vi "Dashboard Main.vi"() -> ()   [LabVIEW 2020]
uses:
  <vilib>/event_ctls.llb/eventvkey.ctl
  <vilib>/Rock Robotics/Network Tables/NT Read Numeric Array.vi
  <vilib>/Rock Robotics/WPI/Dashboard/WPI_DashboardLogging Global.vi
  <vilib>/Rock Robotics/Network Tables/NT Read Boolean.vi
  <vilib>/Rock Robotics/Network Tables/NT Write Boolean.vi
panel:
  in  "Camera Settings Right":T1={"Frame Rate"=30, "Compression"=30, "Size"=1, "DB Camera Config"=FALSE} {"Frame Rate" scale=1.0..30.0; "Compression" scale=100.0..-1.0; "Size" items=["640x480", "320x240", "160x120"]}
  in  "Camera Name Right":string(combo)="No Camera Selection"
  out "Camera Perf":string
  in  "Camera Settings":T1={"Frame Rate"=30, "Compression"=30, "Size"=1, "DB Camera Config"=FALSE} {"Frame Rate" scale=1.0..30.0; "Compression" scale=100.0..-1.0; "Size" items=["640x480", "320x240", "160x120"]}
  in  "TCP":refnum<k5>
  in  "Rec Mode":enum32{"Stop", "Record", "Playback"}(radio)
  out "Robot IP":string
  out "Image Message":string="Timeout in Camera Communications"
  in  "Dashboard Tab":T2(tab)=enum."Custom"
  in  "Select Auto":string(combo)="Select Autonomous ..."
  out "NT Connection":bool
  out "MotorChart R":cluster{"Numeric":dbl, "Numeric":dbl}(graph)
  out "MotorChart L":cluster{"Numeric":dbl, "Numeric":dbl}(graph)
  out "MotorSliders R":cluster{"MotorSlide1":dbl, "MotorSlide2":dbl} {"MotorSlide2" scale=-1.0..1.0 scale format="%#_2e"; "MotorSlide1" scale=-1.0..1.0 scale format="%#_2e"}
  out "MotorSliders L":cluster{"MotorSlide1":dbl, "MotorSlide2":dbl} {"MotorSlide2" scale=-1.0..1.0 scale format="%#_2e"; "MotorSlide1" scale=-1.0..1.0 scale format="%#_2e"}
  out "Gyro":dbl(knob) scale=0.0..360.0
  out "JS1 Z":dbl(slide) scale=-1.0..1.0 scale format="%#_2e"
  out "JS1 Graph":cluster{"X":dbl, "Y":dbl}[](graph)
  out "JS1 Buttons":T3
  out "JS2 Z":dbl(slide) scale=-1.0..1.0 scale format="%#_2e"
  out "JS2 Graph":cluster{"X":dbl, "Y":dbl}[](graph)
  out "JS2 Buttons":T3
  out "Mode":T4(ring)=enum."Auto Disabled"
  out "Right Camera Perf":cluster{"Bandwidth (Mbps)":dbl, "FPS":dbl}
  out "Camera Image Right":T5(plugin-control)
  in  "DB/String 9":string
  in  "DB/String 8":string
  in  "DB/String 7":string
  in  "DB/String 6":string
  in  "DB/String 5":string
  in  "DB/String 4":string
  in  "DB/String 3":string
  in  "DB/String 2":string
  in  "DB/String 1":string
  in  "DB/String 0":string
  in  "DB/Slider 0":dbl(slide) scale=0.0..5.0
  in  "DB/Slider 1":dbl(slide) scale=0.0..5.0
  in  "DB/Slider 2":dbl(slide) scale=0.0..5.0
  in  "DB/Slider 3":dbl(slide) scale=0.0..5.0
  out "DB/LED 3":bool
  out "DB/LED 2":bool
  out "DB/LED 1":bool
  out "DB/LED 0":bool
  in  "DB/Button 3":bool
  in  "DB/Button 2":bool
  in  "DB/Button 1":bool
  in  "DB/Button 0":bool caption="New Name"
  in  "Y2":dbl
  in  "Y1":dbl
  in  "X2":dbl
  in  "X1":dbl
  in  "BasicSpool":dbl
  in  "BasicArm":dbl
  in  "DforTSpeed":dbl
  in  "MobilityD":dbl
  in  "True = facing nodes\nFalse = not":bool=TRUE
  in  "Hybrid":bool
  in  "Mobility?":bool
  in  "Cone?":bool
  in  "offset":dbl
  in  "True = High\nFalse = Low":bool
  in  "Node#":dbl
  in  "True = Blue\nFalse  = Red":bool
  out "Transmit FiFo count":dbl
  out "BusOffCount":dbl
  out "Transmit Err":dbl
  out "Err count":dbl
  out "Util%":dbl
  in  "Auto Delay":dbl
  out "Back right":dbl
  out "Back left":dbl
  out "Front right":dbl
  out "Front left":dbl
  out "Navx connected":bool
  out "yaw":dbl
  in  "Test Slider":dbl(slide) scale=0.0..100.0 scale format="%#_3g"
  in  "On/Off":bool caption="Solenoid"
  in  "Test Name":u16(ring) items=["Select the test to run..."]
  in  "Test Tree":string(tree)
  in  "Motor":cluster{"Value":dbl, "Enable":bool} {"Value" scale=-1.0..1.0 scale format="%#_3g"}
  out "Progress":T6 {"Test Progress" scale=0.0..100.0}
  in  "Rev/Fwd":cluster{"Forward":bool, "Reverse":bool}
  in  "Test Ring":u16(ring) items=["Monochrome", "Color"]
  in  "CheckList":i32(listbox)
  out "Tree":string(tree)
  out "Camera Image":T5(plugin-control)
  out "Background":bool
  in  "Camera Name":string(combo)="No Camera Selection"
  # "HW"
  # "HW"
  # "Joysticks"
  # "Drive Motors"
  # "Front"
  # "Right"
  # "Left"
  # "Back"
  # "AUTO"
  # "CAN stuff"
  # "POINTS FOR PLOTPURSUIT"
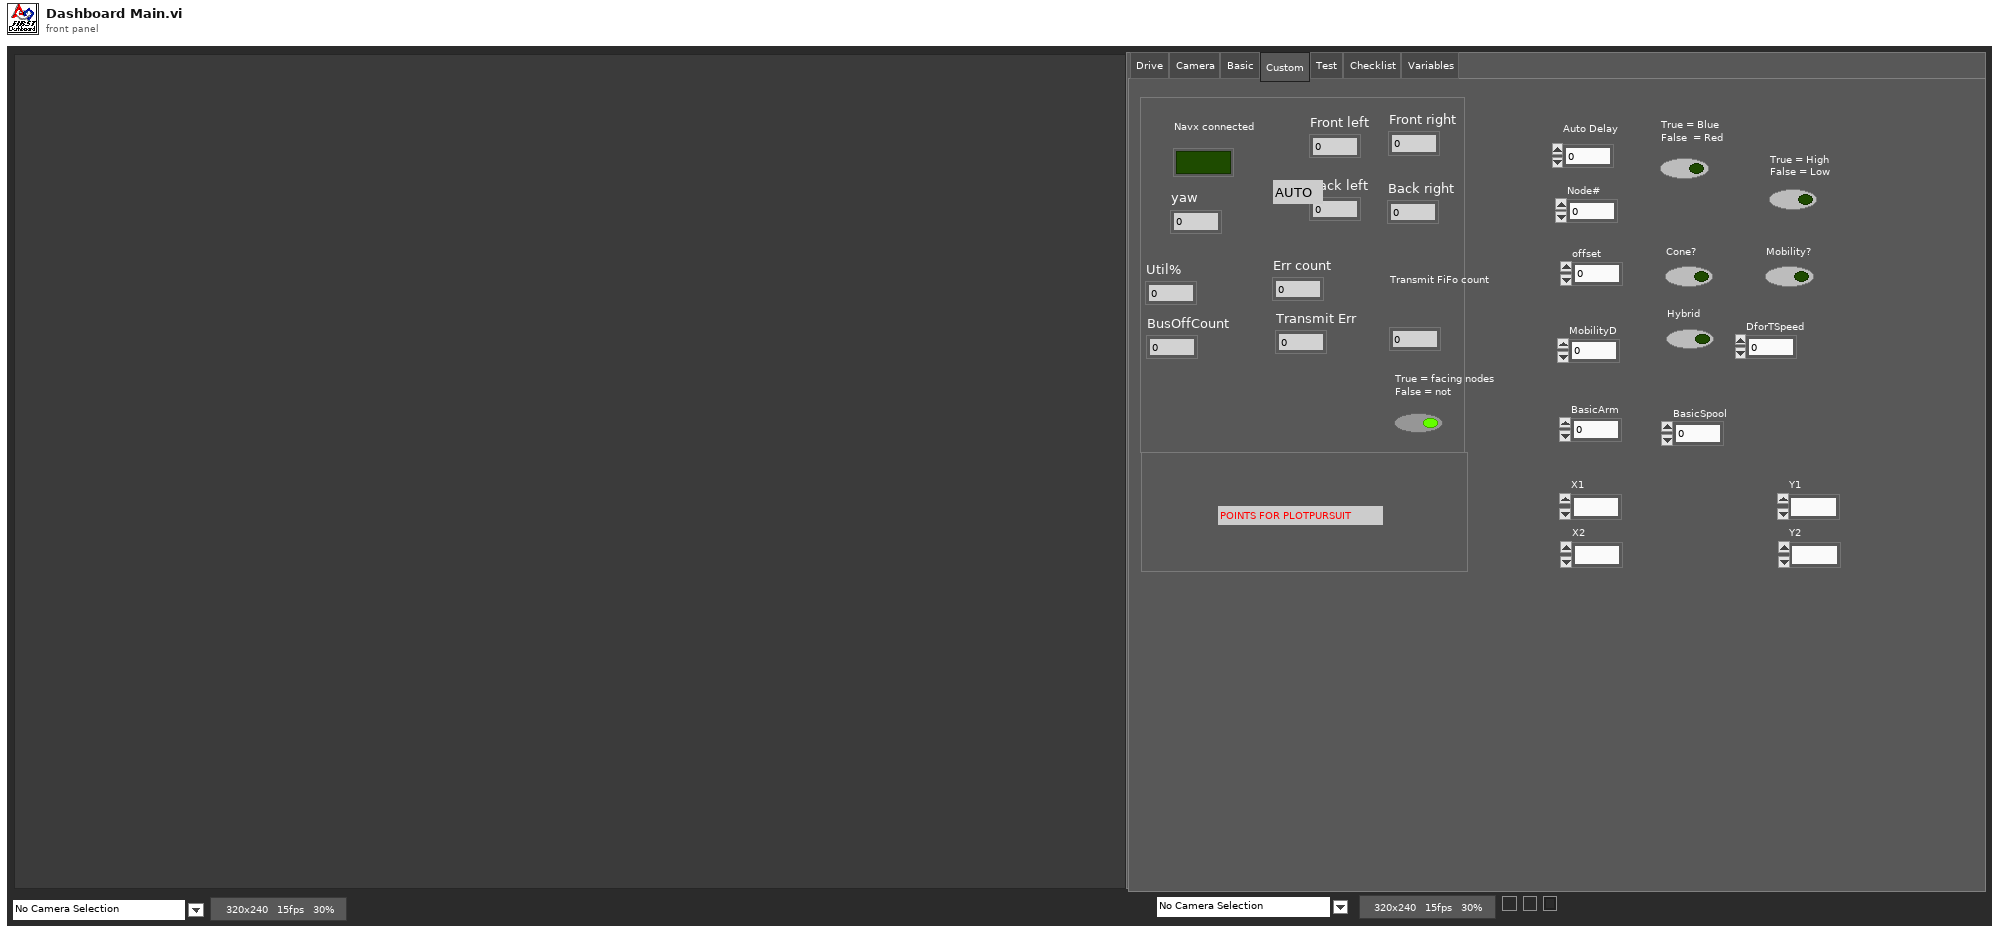
[diagram p1: front panel]
types:
  T1 = cluster{"Frame Rate":i32, "Compression":i32, "Size":u16, "DB Camera Config":bool}
  T2 = enum32{"Drive", "Camera", "Basic", "Custom", "Test", "Checklist", "Variables"}
  T3 = cluster{bool, bool, bool, bool, bool, bool, bool, bool, bool, bool, bool, bool}
  T4 = enum8{"Tele-Op Disabled", "Tele-Op Enabled", "Auto Disabled", "Auto Enabled", "Test Disabled", "Test Enabled", "Disconnected", "No Code", "E-Stop"}
  T5 = typedef "IMAQ Image.ctl" = refnum<image>
  T6 = cluster{"Test Progress":u8, "Test Progress Text":string}
  T7 = cluster{"Save Path":path, "Interval (s)":dbl, "Keep":i32}
  T8 = enum32{"Drive", "Camera", "Basic", "Custom", "Test", "Commands", "Checklist", "Variables"}
  T9 = typedef "Image Type" = u32
  T10 = cluster{"Camera Image":refnum<vi>, "Dashboard Tab":refnum<vi>, "Background":refnum<vi>, "Rec Mode":refnum<vi>, "Test Slider":refnum<vi>, "On/Off ":refnum<vi>, "Test Ring":refnum<vi>, "Rev/Fwd":refnum<vi>, "Test Name":refnum<vi>, "Motor":refnum<vi>, "Progress":refnum<vi>, "CheckList":refnum<vi>, "Tree":refnum<vi>, "Test Tree":refnum<vi>, "Camera Settings":refnum<vi>, "Camera Name":refnum<vi>, "Camera Perf":refnum<vi>, "Camera Settings Right":refnum<vi>, "Camera Name Right":refnum<vi>, "Camera Image Right":refnum<vi>}
  T11 = cluster{"Global Rectangle":i32[], "Contours":cluster{"Contour Type":u32, "ROI Type":u32, "Points":i32[]}[]}
  T12 = cluster{"Camera Name Right":string, string, "Saved DB Images Info":cluster{"Save Path":path, "Interval (s)":dbl, "Keep":i32}}
  T13 = cluster{"Operation":enum16{"Update", "Clear"}, "Color Box":u32}[]
  T14 = typedef "eventvkey.ctl" = enum16{"ASCII", "Enter", "Return", "Shift", "Ctrl", "Alt", "Cmd", "Opt", "Caps", "NumLock", "Clear", "Break", "Up", "Down", "Left", "Right", "Insert", "Delete", "Home", "End", "PageUp", "PageDown", "Escape", "Help", "Pause", "ScrollLock", "F1", "F2", "F3", "F4", "F5", "F6", "F7", "F8", "F9", "F10", "F11", "F12", "F13", "F14", "F15", "F16", "F17", "F18", "F19", "F20", "F21", "F22", "F23", "F24", "Play", "VolumeUp", "VolumeDown", "Mute", "Two Byte Char"}
  T15 = cluster{"Image Size":bool, "Image Type":bool, "Pixel Value":bool, "ROI Information":bool, "Zoom Factor":bool}
  T16 = cluster{"Operation":enum16{"Update", "Clear"}, "Color Box":u32}
  T17 = cluster{"Shift":bool, "Ctrl":bool, "Alt":bool, "Cmd":bool, "Opt":bool}
  T18 = cluster{"Error Strings":string, "Disable Counts":cluster{u16, u16}, "Rail Faults":cluster{u16, u16, u16}, "Robot IP":string, "DB Mode":u8, "Event Info":cluster{"Name":string, "Type":u8, "Number":u16, "Replay":u8}}
  T19 = cluster{"Storage":cluster{"Disk Free":u64, "RAM Block":u32, "RAM free":u32}, "CPU Utilization":cluster{"CPU % ISR":sgl, "CPU % Time Crit":sgl, "CPU % Timed Str":sgl, "CPU % High":sgl, "CPU % Above":sgl, "CPU % Normal":sgl, "CPU % Low":sgl}, "CAN":cluster{"% Bus Utilization":sgl, "Bus Off Cnt":u32, "TX_FIFO Full Cnt":u32, "Receive Error Cnt":u8, "Transmit Error Cnt":u8}, "HID":cluster{"HID Outputs":u32, "Rumble Low":u16, "Rumble High":u16}[]}
  T20 = cluster{"Status bits":cluster{"Test Mode":bool, "Autonomous":bool, "Enabled":bool, "Code Start":bool, "Brownout":bool, "Reserved 2":bool, "Reserved 3":bool, "E-Stop":bool}, "Code Trace":cluster{"Disabled":bool, "TeleOp":bool, "Auto":bool, "Test":bool}, "Controller Type":enum16{"unknown", "cRIO", "roboRio"}, "Code?":enum16{"unknown", "noCode", "code"}, "Battery V":dbl}
  T21 = cluster{"Control Bits":cluster{"TestMode":bool, "Autonomous":bool, "Enabled":bool, "FMS Present":bool, bool, bool, bool, "E-Stop":bool}, "Team Station ":u8, "Countdown":sgl, "Joystick Values":cluster{"Axes":dbl[], "Buttons":bool[], "POVs":i16[]}[]}
  T22 = cluster{"Axes":dbl[], "Buttons":bool[], "POVs":i16[]}[]
  T23 = cluster{"Axes":dbl[], "Buttons":bool[], "POVs":i16[]}
  T24 = cluster{"Buttons[0]":bool, "Buttons[1]":bool, "Buttons[2]":bool, "Buttons[3]":bool, "Buttons[4]":bool, "Buttons[5]":bool, "Buttons[6]":bool, "Buttons[7]":bool, "Buttons[8]":bool, "Buttons[9]":bool, "Buttons[10]":bool, "Buttons[11]":bool}
  T25 = cluster{"Camera Name":string, string, "Saved DB Images Info":cluster{"Save Path":path, "Interval (s)":dbl, "Keep":i32}}
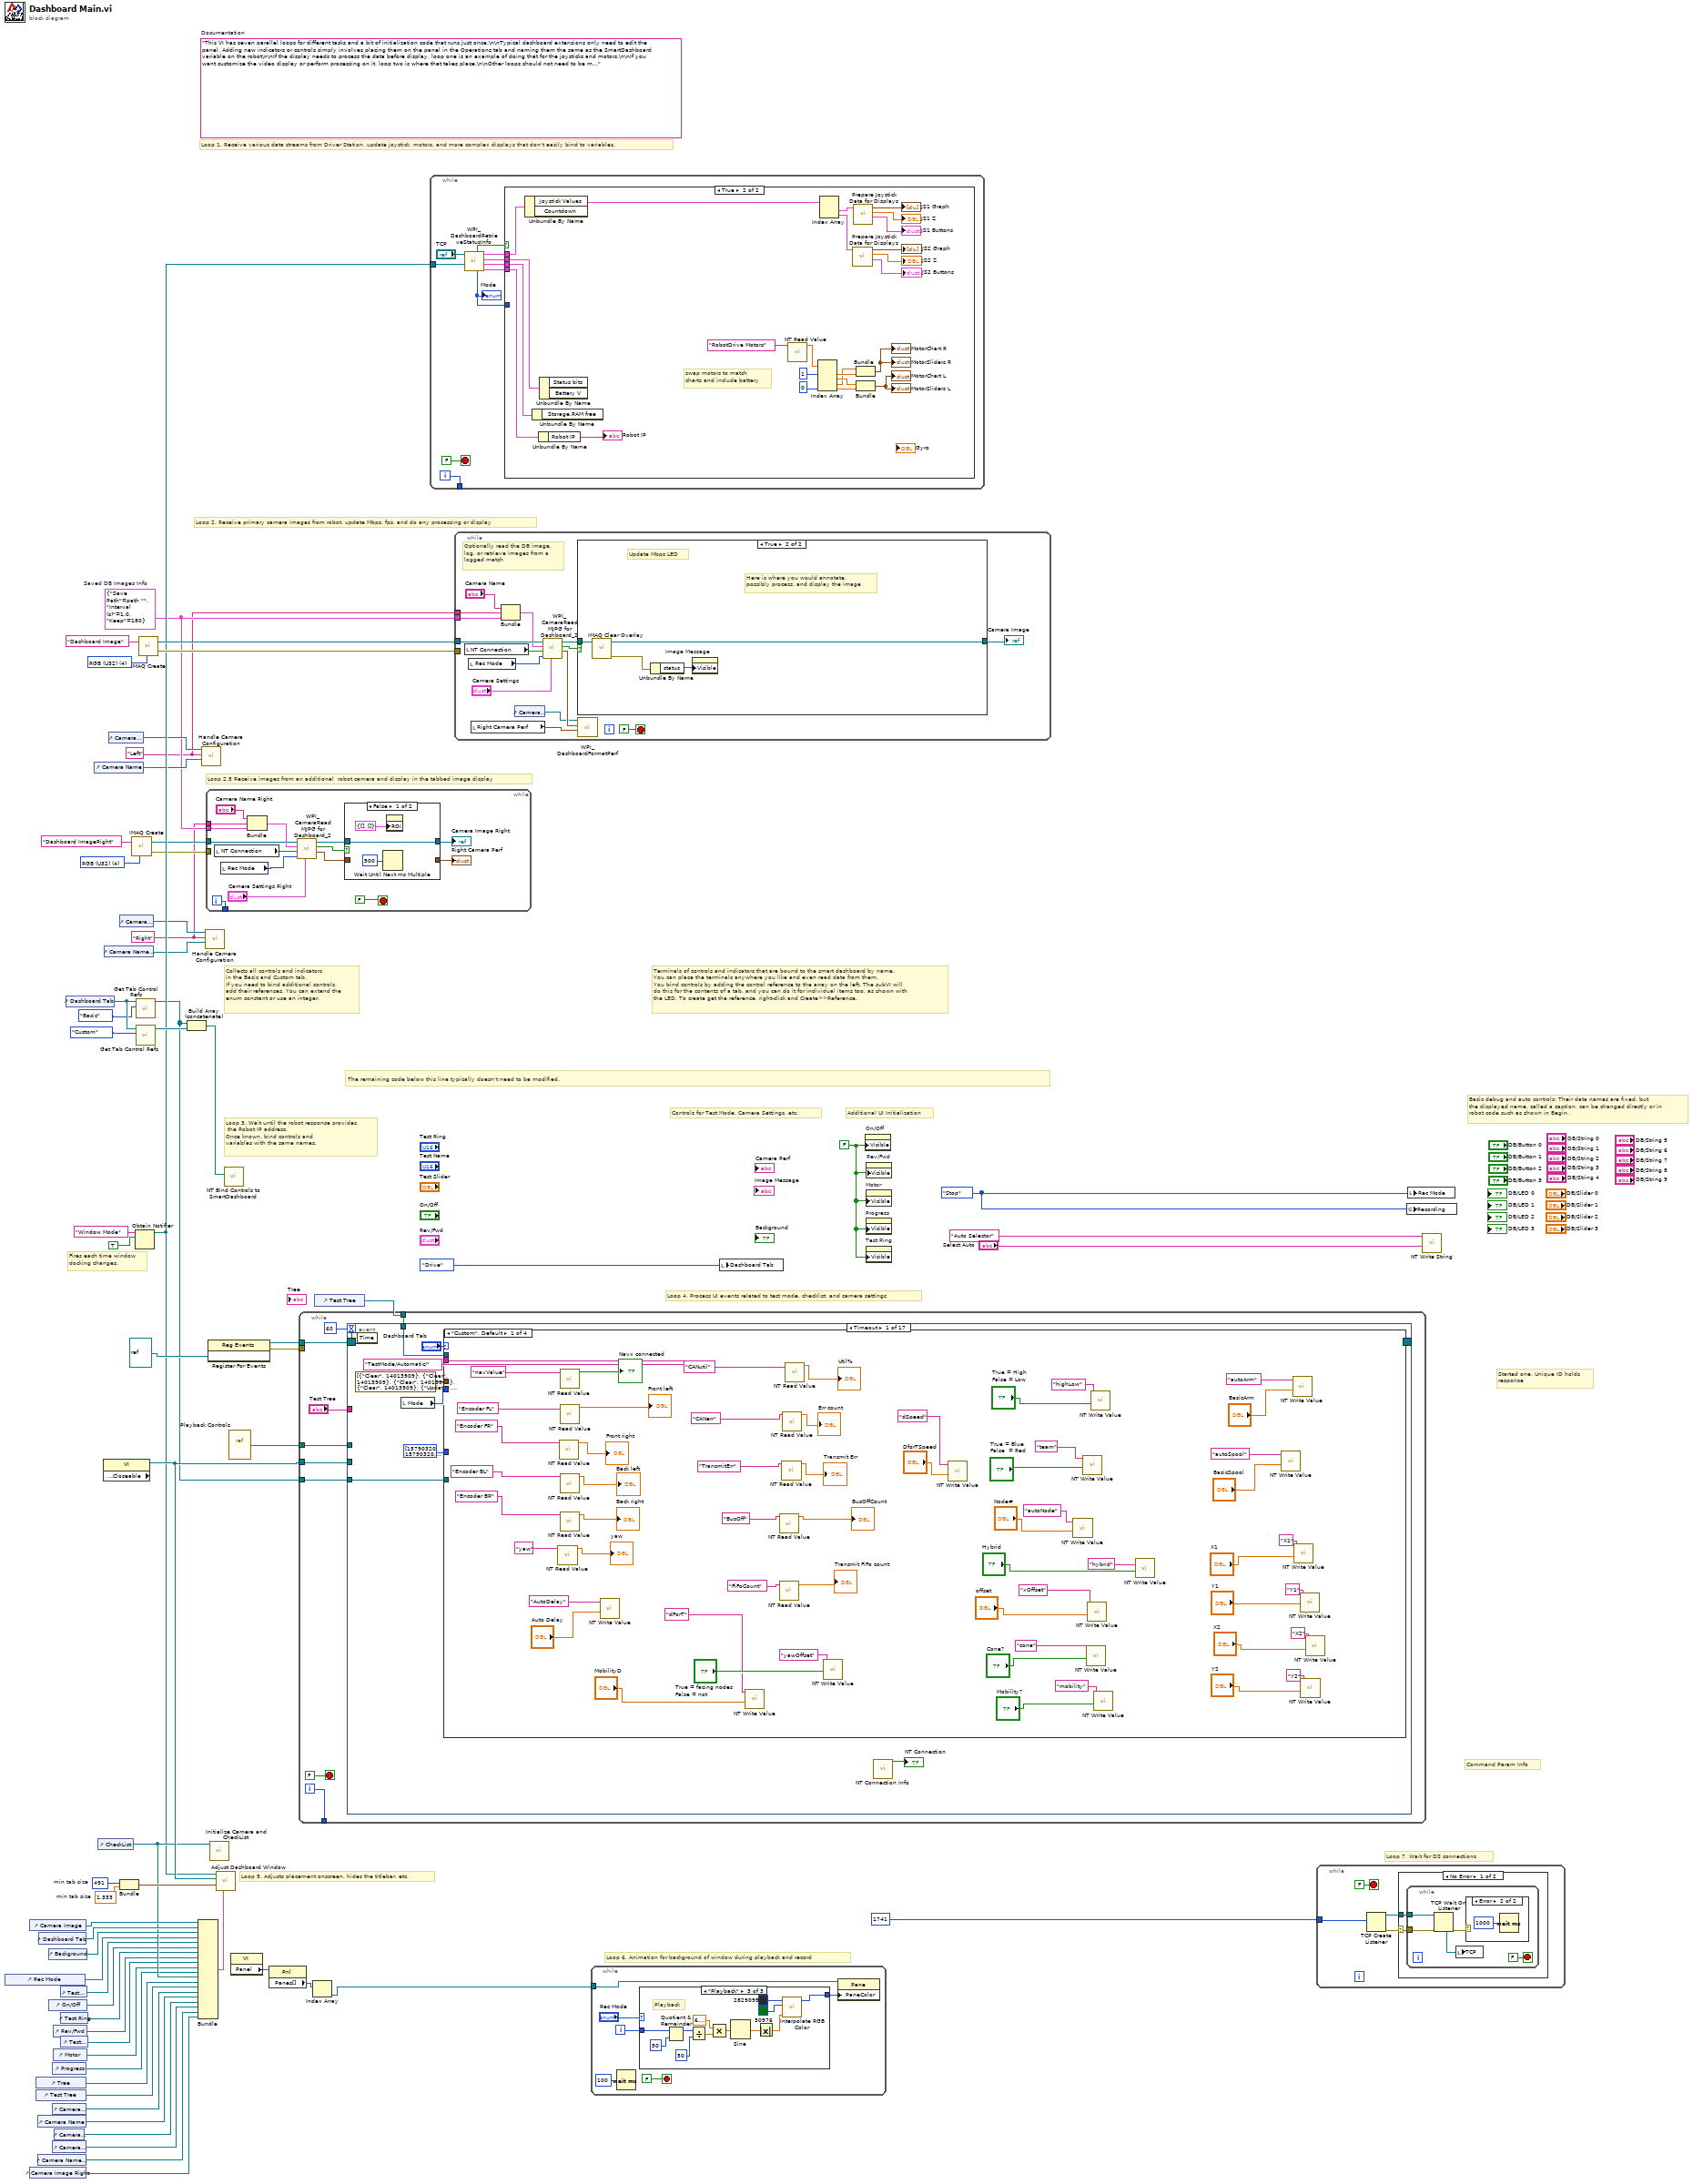
[diagram p0: block diagram]
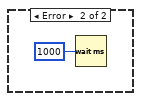
[diagram p4: hidden frame]
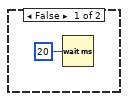
[diagram p5: hidden frame]
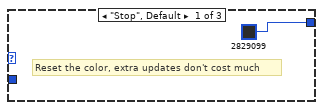
[diagram p6: hidden frame]
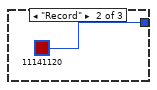
[diagram p7: hidden frame]
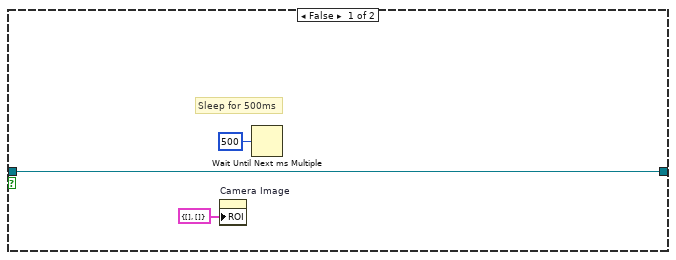
[diagram p8: hidden frame]
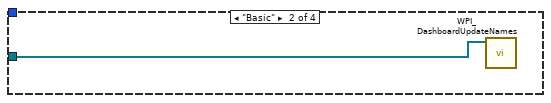
[diagram p9: hidden frame]
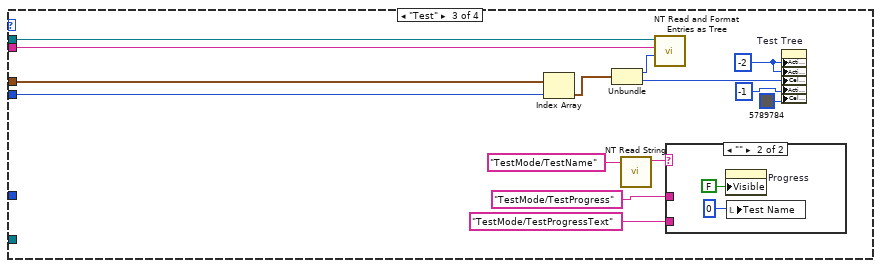
[diagram p10: hidden frame]
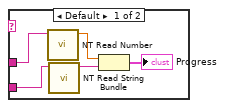
[diagram p11: hidden frame]
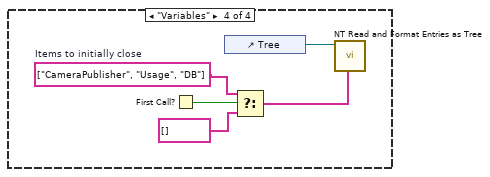
[diagram p12: hidden frame]
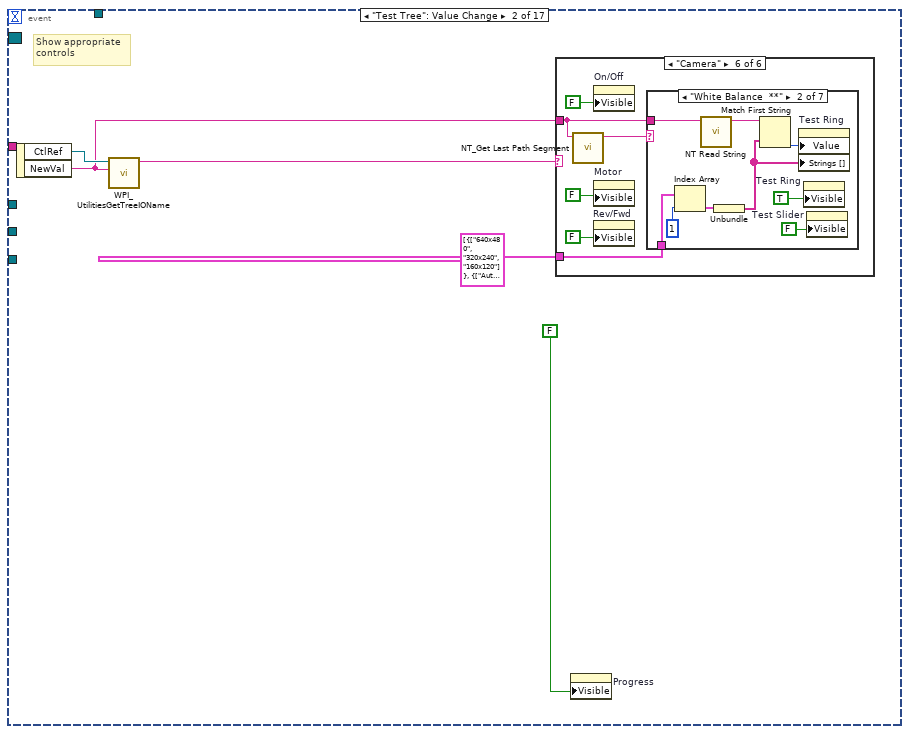
[diagram p13: hidden frame]
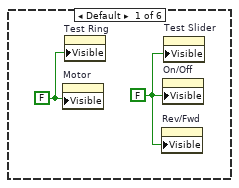
[diagram p14: hidden frame]
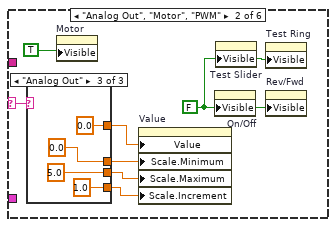
[diagram p15: hidden frame]
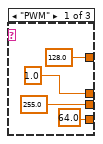
[diagram p16: hidden frame]
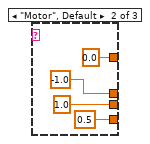
[diagram p17: hidden frame]
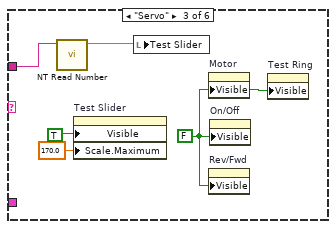
[diagram p18: hidden frame]
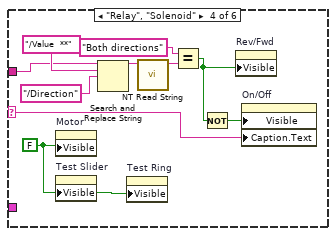
[diagram p19: hidden frame]
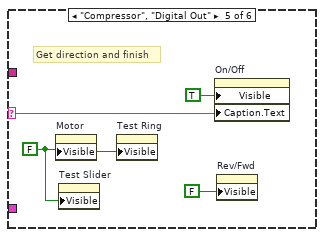
[diagram p20: hidden frame]
diagram:
  w3 = T7 {"Save Path"=path "", "Interval (s)"=1.0, "Keep"=180}  # Saved DB Images Info
  w2 = "Right"
  w1 = "Left"
  w13 = T9 4 items=["Grayscale (U8)", "Grayscale (I16)", "Grayscale (SGL)", "Complex (CSG)", "RGB (U32)", "HSL (U32)", "RGB (U64)"] ("Image Type")
  w42 = 491  # min tab size
  w41 = 1.333  # min tab size
  w49 = enum32{"Stop", "Record", "Playback"}."Stop" ("Rec Mode")
  w26 = FALSE ("Visible")
  (unwired) "This VI has seven parallel loops for different tasks and a bit of initialization code that runs just once.\n\nTypical dashboard extensions only need to edit the panel. Adding new indicators or controls simply involves placing them on the panel in the Operations tab and naming them the same as the SmartDashboard variable on the robot\n\nIf the display needs to process the data before display, loop one is an example of doing that for the joysticks and motors.\n\nIf you want customize the video display or perform processing on it, loop two is where that takes place.\n\nOther loops should not need to be modified. They are pretty standard, and document the task they perform."  # Documentation
  w63 = T9 4 items=["Grayscale (U8)", "Grayscale (I16)", "Grayscale (SGL)", "Complex (CSG)", "RGB (U32)", "HSL (U32)", "RGB (U64)"] ("Image Type")
  # "Loop 2.5 Receive images from an additional  robot camera and display in the tabbed image display"
  # "Command Param Info"
  # "Started one, Unique ID holds\nresponse"
  # "Loop 7. Wait for DS connections"
  # "Basic debug and auto controls: Their data names are fixed, but\nthe displayed name, called a caption, can be changed directly or in\nrobot code such as shown in Begin."
  # "Controls for Test Mode, Camera Settings, etc."
  # "Additional UI Initialization"
  # "Loop 6. Animation for background of window during playback and record"
  # "Fires each time window\ndocking changes."
  # "Collects all controls and indicators\nin the Basic and Custom tab.\nIf you need to bind additional controls,\nadd their references. You can extend the\nenum constant or use an integer."
  # "The remaining code below this line typically doesn't need to be modified."
  # "Loop 4. Process UI events related to test mode, checklist, and camera settings"
  # "Terminals of controls and indicators that are bound to the smart dashboard by name.\nYou can place the terminals anywhere you like and even read data from them.\nYou bind controls by adding the control reference to the array on the left. The subVI will\ndo this for the contents of a tab, and you can do it for individual items too, as shown with\nthe LED. To create get the reference, right-click and Create>>Reference."
  # "Loop 3. Wait until the robot response provides\n the Robot IP address.\nOnce known, bind controls and\nvariables with the same names."
  # "Loop 5. Adjusts placement onscreen, hides the titlebar, etc."
  # "Loop 1. Receive various data streams from Driver Station, update joystick, motors, and more complex displays that don't easily bind to variables."
  # "Loop 2. Receive primary camera images from robot, update Mbps, fps, and do any processing or display"
  n1 = control-ref of="Rec Mode"() -> (w32:refnum<vi>)
  n2 = control-ref of="Camera Image Right"() -> (w6:refnum<vi>)
  n3 = control-ref of="Camera Image"() -> (w44:refnum<vi>)
  n4 = control-ref of="Tree"() -> (w36:refnum<vi>)
  n5 = control-ref of="Test Tree"() -> (w35:refnum<vi>)
  n6 = control-ref of="Camera Name"() -> (w19:refnum<vi>)
  n7 = control-ref of="Camera Name Right"() -> (w7:refnum<vi>)
  n8 = control-ref of="Dashboard Tab"() -> (w43:refnum<vi>)
  n9 = control-ref of="Background"() -> (w39:refnum<vi>)
  n10 = control-ref of="On/Off"() -> (w30:refnum<vi>)
  n11 = control-ref of="Progress"() -> (w27:refnum<vi>)
  n12 = control-ref of="Camera Settings"() -> (w20:refnum<vi>)
  n13 = control-ref of="Camera Settings Right"() -> (w8:refnum<vi>)
  n14 = control-ref of="Rev/Fwd"() -> (w28:refnum<vi>)
  n15 = control-ref of="Motor"() -> (w33:refnum<vi>)
  n16 = control-ref of="Camera Perf"() -> (w18:refnum<vi>)
  n17 = control-ref of="Test Slider"() -> (w31:refnum<vi>)
  n18 = control-ref of="Test Ring"() -> (w29:refnum<vi>)
  n19 = control-ref of="Test Name"() -> (w34:refnum<vi>)
  n20 = control-ref of="Dashboard Tab"() -> (w47:refnum<vi>)
  n21 = control-ref of="Camera Name"() -> (w21:refnum<vi>)
  n22 = control-ref of="CheckList"() -> (w37:refnum<vi>)
  n23 = property class="VI" props=["Front Panel.Closeable"]() -> (reference out=w48:refnum<vi>)  [unwired: 2 in, 2 out]
  n24 = control-ref of="Camera Name Right"() -> (w9:refnum<vi>)
  n25 = control-ref of="Camera Settings"() -> (w22:refnum<vi>)
  n26 = control-ref of="Camera Settings Right"() -> (w10:refnum<vi>)
  n27 = Bundle("min tab size"=w42, "min tab size"=w41) -> (w40:cluster{"min tab size":i32, "min tab size":dbl})  [unwired: 1 in]
  n28 = call "IMAQ Create"("Image Name"="Dashboard ImageRight", "Image Type"=w13) -> ("New Image"=w12:T5, "error out"=w11:errorcluster)  [unwired: 2 in, 1 out]
  n29 = Obtain Notifier(name (unnamed)="Window Mode", notification data type=TRUE) -> (notifier out=w25:refnum<notifier>)  [unwired: 2 in, 2 out]
  n30 = call <vilib>:"Get Tab Control Refs.vi"("Page Index"=T8."Basic" ("Dashboard Tab"), "TabControl in"=w47) -> ("ControlsOnPage"=w17:refnum<vi>[])  [unwired: 9 in]
  n31 = call <vilib>:"Get Tab Control Refs.vi"("Page Index"=T8."Custom" ("Dashboard Tab"), "TabControl in"=w47) -> ("ControlsOnPage"=w46:refnum<vi>[])  [unwired: 9 in]
  n32 = call "IMAQ Create"("Image Name"="Dashboard Image", "Image Type"=w63) -> ("New Image"=w61:T5, "error out"=w60:errorcluster)  [unwired: 2 in, 1 out]
  n33 = Build Array (concatenate)(w17, w46) -> (w45:refnum<vi>[])
  n34 = Bundle("Camera Image"=w44, "Dashboard Tab"=w43, "Background"=w39, "Rec Mode"=w32, "Test Slider"=w31, "On/Off"=w30, "Test Ring"=w29, "Rev/Fwd"=w28, "Test Name"=w34, "Motor"=w33, "Progress"=w27, "CheckList"=w37, "Tree"=w36, "Test Tree"=w35, "Camera Settings"=w20, "Camera Name"=w19, "Camera Perf"=w18, "Camera Settings Right"=w8, "Camera Name Right"=w7, "Camera Image Right"=w6) -> (w38:T10)  [unwired: 1 in]
  n35 = call "Handle Camera Configuration.vi"("CameraNameRef"=w21, "Display Name"=w1, "ClusterRef"=w22) -> ()  [unwired: 9 in]
  n36 = call "Handle Camera Configuration.vi"("CameraNameRef"=w9, "Display Name"=w2, "ClusterRef"=w10) -> ()  [unwired: 9 in]
  n37 = while {
    tunnel: w12 -> [w78]
    tunnel: w11 -> [_]
    tunnel: [w73] -> _
    tunnel: w3 -> [w69]
    tunnel: w2 -> [w66]
    i -> [w73]
    stop <- FALSE stop-if-true
    n38 = local read "NT Connection"() -> (w70:bool)
    n39 = local read "Rec Mode"() -> (w77:enum32{"Stop", "Record", "Playback"})
    n40 = Bundle("Camera Name Right"="Camera Name Right", w66, "Saved DB Images Info"=w69) -> (w68:T12)  [unwired: 1 in]
    n41 = call <vilib>:"WPI_CameraRead MJPG for Dashboard_2.vi"("Camera Settings"="Camera Settings Right", "Rec Mode"=w77, "NT Connection"=w70, "Capture Info"=w68, "Image in"=w78) -> ("perf info"=w64:cluster{"Bandwidth (Mbps)":dbl, "fps":dbl}, "Active"=w72:bool, "Image\\ out"=w75:T5)  [unwired: 4 in]
    n42 = case shown="False" w72 {
      tunnel: w75 -> [w80 w83]
      tunnel: [w80 w83] -> w71
      tunnel: [_ w82] -> w65
      tunnel: w64 -> [_ w82]
      frame False {
        n43 = Wait Until Next ms Multiple(millisecond multiple=u32 500) -> ()  [unwired: 1 out]
        n44 = property on="Camera Image Right" class="ImageControl"("ROI"=T11 {"Global Rectangle"=[], "Contours"=[]}) -> ()  [unwired: 2 in, 2 out]
      }
      frame True {
      }
    }
    "Camera Image Right" <- w71
    "Right Camera Perf" <- w65
  }
  n45 = register-events(refnum<vi> refnum) -> (reference out=w52:refnum<event-registration>, error out=w51:errorcluster)  [unwired: 2 in]
  n46 = call "Initialize Camera and CheckList.vi"("ListBox in"=w37) -> ()  [unwired: 11 in]
  n47 = call "Adjust Dashboard Window.vi"("Sizing Refnums"=w38, "Size Constraints"=w40, "VI"=w48, "WIn Mode"=w25) -> ()  [unwired: 8 in]
  n48 = call <vilib>:"NT Bind Controls to SmartDashboard.vi"("Bound Control Refs"=w45) -> ()  [unwired: 11 in]
  n49 = vi-ref "Playback Controls.vi"() -> (w53:refnum<vi>)
  n50 = property class="VI"() -> ("Panel"=w55:refnum<vi>)  [unwired: 2 in, 2 out]
  n51 = property class="Pnl"(reference=w55) -> ("Panes[]"=w56:refnum<vi>[])  [unwired: 1 in, 2 out]
  n52 = Index Array(array=w56) -> (element=w54:refnum<vi>)  [unwired: 1 in]
  n53 = control-ref of="Test Tree"() -> (w57:refnum<vi>)
  n54 = while {
    tunnel: [w89] -> _
    tunnel: w57 -> [w88]
    tunnel: w53 -> [w87]
    tunnel: w52 -> [w86]
    tunnel: w51 -> [_]
    tunnel: w48 -> [w85]
    tunnel: w17 -> [w84]
    i -> [w89]
    stop <- FALSE stop-if-true
    n55 = event shown="[0] Timeout" {
      selector: w86 -> [_ _ _ _ _ _ _ _ _ _ _ _ _ _ _ _ _]
      dyn-events: [_ _ _ _ _ _ _ _ _ _ _ _ _ w350 _ _ _] -> _
      timeout: u32 60 ("milliseconds to wait") -> [_ _ _ _ _ _ _ _ _ _ _ _ _ _ _ _ _]
      tunnel: w88 -> [w99 _ _ _ _ _ _ _ _ _ _ _ _ _ _ _ _]
      tunnel: "Test Tree" -> [_ _ _ _ _ _ _ _ w323 w330 w331 w334 w341 _ _ _ _]
      tunnel: w87 -> [_ _ _ _ _ _ _ _ _ _ _ _ _ w352 _ w367 _]
      tunnel: w85 -> [_ _ _ _ _ _ _ _ _ _ _ _ _ w348 _ _ _]
      tunnel: w84 -> [w94 _ _ _ _ _ _ _ _ _ _ _ _ _ _ _ _]
      event Timeout {
        n56 = event-data() -> ()  [unwired: 1 in, 1 out]
        n57 = local read "Mode"() -> (w97:T4)
        n58 = case shown="\"Custom\", Default" "Dashboard Tab" {
          tunnel: w99 -> [_ _ w171 _]
          tunnel: "TestMode/Automatic/" ("Name Pattern") -> [_ _ w170 _]
          tunnel: T13 [{"Operation"=enum."Clear", "Color Box"=14013909}, {"Operation"=enum."Clear", "Color Box"=14013909}, {"Operation"=enum."Clear", "Color Box"=14013909}, {"Operation"=enum."Clear", "Color Box"=14013909}, {"Operation"=enum."Update", "Color Box"=14013909}, {"Operation"=enum."Update", "Color Box"=16777215}, {"Operation"=enum."Clear", "Color Box"=14013909}, {"Operation"=enum."Clear", "Color Box"=14013909}, {"Operation"=enum."Clear", "Color Box"=14013909}] -> [_ _ w163 _]
          tunnel: w97 -> [_ _ w162 _]
          tunnel: u32[] [15790320, 15790320, 15790320, 15790320, 16777215, 16777215, 15790320, 15790320, 15790320] -> [_ _ _ _]
          tunnel: w94 -> [_ w157 _ _]
          frame "Custom", Default {
            n59 = call-poly <vilib>:"NT Read Value.vi"("name"="yaw") -> ("value"=→"yaw":dbl)  [unwired: 8 in, 2 out]
            n60 = call-poly <vilib>:"NT Read Value.vi"("name"="Encoder FR") -> ("value"=→"Front right":dbl)  [unwired: 8 in, 2 out]
            n61 = call-poly <vilib>:"NT Read Value.vi"("name"="navValue") -> ("value"=→"Navx connected":bool)  [unwired: 8 in, 2 out]
            n62 = call-poly <vilib>:"NT Read Value.vi"("name"="Encoder BL") -> ("value"=→"Back left":dbl)  [unwired: 8 in, 2 out]
            n63 = call-poly <vilib>:"NT Read Value.vi"("name"="Encoder BR") -> ("value"=→"Back right":dbl)  [unwired: 8 in, 2 out]
            n64 = call-poly <vilib>:"NT Read Value.vi"("name"="Encoder FL") -> ("value"=→"Front left":dbl)  [unwired: 8 in, 2 out]
            n65 = call-poly <vilib>:"NT Write Value.vi"("value"="Auto Delay", "name"="AutoDelay") -> ()  [unwired: 9 in, 1 out]
            n66 = call-poly <vilib>:"NT Write Value.vi"("value"="MobilityD", "name"="dForT") -> ()  [unwired: 9 in, 1 out]
            n67 = call-poly <vilib>:"NT Read Value.vi"("name"="BusOff") -> ("value"=→"BusOffCount":dbl)  [unwired: 8 in, 2 out]
            n68 = call-poly <vilib>:"NT Read Value.vi"("name"="FiFoCount") -> ("value"=→"Transmit FiFo count":dbl)  [unwired: 8 in, 2 out]
            n69 = call-poly <vilib>:"NT Read Value.vi"("name"="TransmitErr") -> ("value"=→"Transmit Err":dbl)  [unwired: 8 in, 2 out]
            n70 = call-poly <vilib>:"NT Read Value.vi"("name"="CANerr") -> ("value"=→"Err count":dbl)  [unwired: 8 in, 2 out]
            n71 = call-poly <vilib>:"NT Read Value.vi"("name"="CANutil") -> ("value"=→"Util%":dbl)  [unwired: 8 in, 2 out]
            n72 = call-poly <vilib>:"NT Write Value.vi"("value"="True = facing nodes\nFalse = not", "name"="yawOffset") -> ()  [unwired: 9 in, 1 out]
            n73 = call-poly <vilib>:"NT Write Value.vi"("value"="DforTSpeed", "name"="dSpeed") -> ()  [unwired: 9 in, 1 out]
            n74 = call-poly <vilib>:"NT Write Value.vi"("value"="Node#", "name"="autoNode") -> ()  [unwired: 9 in, 1 out]
            n75 = call-poly <vilib>:"NT Write Value.vi"("value"="True = Blue\nFalse  = Red", "name"="team") -> ()  [unwired: 9 in, 1 out]
            n76 = call-poly <vilib>:"NT Write Value.vi"("value"="Cone?", "name"="cone") -> ()  [unwired: 9 in, 1 out]
            n77 = call-poly <vilib>:"NT Write Value.vi"("value"="offset", "name"="xOffset") -> ()  [unwired: 9 in, 1 out]
            n78 = call-poly <vilib>:"NT Write Value.vi"("value"="True = High\nFalse = Low", "name"="highLow") -> ()  [unwired: 9 in, 1 out]
            n79 = call-poly <vilib>:"NT Write Value.vi"("value"="Mobility?", "name"="mobility") -> ()  [unwired: 9 in, 1 out]
            n80 = call-poly <vilib>:"NT Write Value.vi"("value"="Hybrid", "name"="hybrid") -> ()  [unwired: 9 in, 1 out]
            n81 = call-poly <vilib>:"NT Write Value.vi"("value"="BasicSpool", "name"="autoSpool") -> ()  [unwired: 9 in, 1 out]
            n82 = call-poly <vilib>:"NT Write Value.vi"("value"="BasicArm", "name"="autoArm") -> ()  [unwired: 9 in, 1 out]
            n83 = call-poly <vilib>:"NT Write Value.vi"("value"="X1", "name"="X1") -> ()  [unwired: 9 in, 1 out]
            n84 = call-poly <vilib>:"NT Write Value.vi"("value"="Y1", "name"="Y1") -> ()  [unwired: 9 in, 1 out]
            n85 = call-poly <vilib>:"NT Write Value.vi"("value"="Y2", "name"="Y2") -> ()  [unwired: 9 in, 1 out]
            n86 = call-poly <vilib>:"NT Write Value.vi"("value"="X2", "name"="X2") -> ()  [unwired: 9 in, 1 out]
          }
          frame "Basic" {
            n87 = call <vilib>:"WPI_DashboardUpdateNames.vi"("Controls on Tab"=w157) -> ()  [unwired: 11 in]
          }
          frame "Test" {
            w169 = -2 ("Active Item:Row Number")
            n88 = Index Array(array=w163, index=w162) -> (element=w164:T16)
            n89 = Unbundle(w164) -> ("Operation"=w165:enum16{"Update", "Clear"}, "Color Box"=w166:u32)
            n90 = call <vilib>:"NT Read String.vi"("name"="TestMode/TestName" ("Name")) -> ("value"=w160:string)  [unwired: 8 in, 2 out]
            n91 = call <vilib>:"NT Read and Format Entries as Tree.vi"("Operation"=w165, "Name Pattern"=w170, "Tree Refnum"=w171) -> ()  [unwired: 7 in, 2 out]
            n92 = case shown="\"\"" w160 {
              tunnel: "TestMode/TestProgress" ("Name") -> [w173 _]
              tunnel: "TestMode/TestProgressText" ("Name") -> [w172 _]
              frame Default {
                n93 = call <vilib>:"NT Read Number.vi"("name"=w173) -> ("value"=w174:dbl)  [unwired: 8 in, 2 out]
                n94 = call <vilib>:"NT Read String.vi"("name"=w172) -> ("value"=w175:string)  [unwired: 8 in, 2 out]
                n95 = Bundle("value"=w174, "value"=w175) -> (→"Progress":cluster{"value":dbl, "value":string})  [unwired: 1 in]
              }
              frame "" {
                n96 = property on="Progress" class="Clust (strict)"("Visible"=FALSE) -> ()  [unwired: 2 in, 2 out]
                n97 = local write "Test Name"(u16 0) -> ()
              }
            }
            n98 = property on="Test Tree" class="Tree (strict)"("Active Item Row Number"=w169, "ActiveColNum"=w169, "CellBG"=w166, "Active Item Row Number"=-1 ("Active Item:Row Number"), "CellBG"=u32 5789784 ("Color Box")) -> ()  [unwired: 2 in, 2 out]
          }
          frame "Variables" {
            w181 = string[] ["CameraPublisher", "Usage", "DB"]  # Items to initially close
            n99 = First Call?() -> (First Call?: T/F=w182:bool)
            n100 = control-ref of="Tree"() -> (w183:refnum<vi>)
            n101 = Select(t=w181, s=w182, f=string[] []) -> (s? t:f=w179:string[])
            n102 = call <vilib>:"NT Read and Format Entries as Tree.vi"("Tags to  Close"=w179, "Tree Refnum"=w183) -> ()  [unwired: 8 in, 2 out]
          }
        }
        n103 = call <vilib>:"NT Connection Info.vi"() -> ("Connected"=→"NT Connection":bool)  [unwired: 11 in]
      }
      event "Test Tree": Value Change {
        # "Show appropriate\ncontrols"
        n104 = event-data() -> ("CtlRef"=w187:refnum<vi>, "NewVal"=w185:string)  [unwired: 1 in]
        n105 = call <vilib>:"WPI_UtilitiesGetTreeIOName.vi"("NewVal"=w185, "TreeControl in"=w187) -> ("I/O Name"=w188:string)  [unwired: 9 in]
        n106 = case shown="\"Camera\"" w188 {
          selector: w188 -> [_ w195 _ w217 w226 _]
          tunnel: w185 -> [_ _ w214 w216 _ w233]
          tunnel: cluster{string[]}[] [{["640x480", "320x240", "160x120"]}, {["Auto", "Fixed indoor", "Fixed outdoor 1", "Fixed outdoor 2", "Fixed fluorescent 1", "Fixed fluorescent 2", "Hold current"]}, {["Auto", "Flicker-free 50 Hz", "Flicker-free 60 Hz", "Hold current"]}, {["None", "Prioritize frame rate", "Prioritize image quality"]}, {["Monochrome", "Color"]}] -> [_ _ _ _ _ w232]
          frame Default {
            w190 = FALSE ("Visible")
            w189 = FALSE ("Visible")
            n107 = property on="Motor" class="Clust (strict)"("Visible"=w189) -> ()  [unwired: 2 in, 2 out]
            n108 = property on="Test Ring" class="Ring (strict)"("Visible"=w189) -> ()  [unwired: 2 in, 2 out]
            n109 = property on="Rev/Fwd" class="Clust (strict)"("Visible"=w190) -> ()  [unwired: 2 in, 2 out]
            n110 = property on="On/Off" class="Bool (strict)"("Visible"=w190) -> ()  [unwired: 2 in, 2 out]
            n111 = property on="Test Slider" class="Slide (strict)"("Visible"=w190) -> ()  [unwired: 2 in, 2 out]
          }
          frame "Analog Out", "Motor", "PWM" {
            w196 = FALSE ("Visible")
            n112 = case shown="\"Analog Out\"" w195 {
              tunnel: [1.0 ("Value") -1.0 ("Value") 0.0 ("Value")] -> w194
              tunnel: [255.0 ("Value") 1.0 ("Value") 5.0 ("Value")] -> w193
              tunnel: [128.0 ("Value") 0.0 ("Value") 0.0 ("Value")] -> w192
              tunnel: [64.0 ("Value") 0.5 ("Value") 1.0 ("Value")] -> w191
              frame "PWM" {
              }
              frame "Motor", Default {
              }
              frame "Analog Out" {
              }
            }
            n113 = property on="Motor" class="Clust (strict)"("Visible"=TRUE) -> ()  [unwired: 2 in, 2 out]
            n114 = property on="Value" class="Slide (strict)"("Value"=w192, "Scale.Minimum"=w194, "Scale.Maximum"=w193, "Scale.Increment"=w191) -> ()  [unwired: 2 in, 2 out]
            n115 = property on="On/Off" class="Bool (strict)"("Visible"=w196) -> ()  [unwired: 2 in, 2 out]
            n116 = property on="Test Slider" class="Slide (strict)"("Visible"=w196) -> ()  [unwired: 2 in, 2 out]
            n117 = property on="Test Ring" class="Ring (strict)"("Visible"=w196) -> ()  [unwired: 2 in, 2 out]
            n118 = property on="Rev/Fwd" class="Clust (strict)"("Visible"=w196) -> ()  [unwired: 2 in, 2 out]
          }
          frame "Servo" {
            w212 = FALSE ("Visible")
            n119 = call <vilib>:"NT Read Number.vi"("name"=w214) -> ("value"=w213:dbl)  [unwired: 8 in, 2 out]
            n120 = property on="Test Slider" class="Slide (strict)"("Visible"=TRUE, "Scale.Maximum"=170.0 ("Scale.Range:Maximum")) -> ()  [unwired: 2 in, 2 out]
            n121 = local write "Test Slider"(w213) -> ()
            n122 = property on="Motor" class="Clust (strict)"("Visible"=w212) -> ()  [unwired: 2 in, 2 out]
            n123 = property on="Rev/Fwd" class="Clust (strict)"("Visible"=w212) -> ()  [unwired: 2 in, 2 out]
            n124 = property on="On/Off" class="Bool (strict)"("Visible"=w212) -> ()  [unwired: 2 in, 2 out]
            n125 = property on="Test Ring" class="Ring (strict)"("Visible"=w212) -> ()  [unwired: 2 in, 2 out]
          }
          frame "Relay", "Solenoid" {
            w215 = FALSE ("Visible")
            n126 = property on="Motor" class="Clust (strict)"("Visible"=w215) -> ()  [unwired: 2 in, 2 out]
            n127 = property on="Test Slider" class="Slide (strict)"("Visible"=w215) -> ()  [unwired: 2 in, 2 out]
            n128 = Search and Replace String(input string=w216, search string="/Value  **", replace string="/Direction") -> (result string=w222:string)  [unwired: 5 in, 3 out]
            n129 = property on="Test Ring" class="Ring (strict)"("Visible"=w215) -> ()  [unwired: 2 in, 2 out]
            n130 = call <vilib>:"NT Read String.vi"("name"=w222) -> ("value"=w220:string)  [unwired: 8 in, 2 out]
            n131 = Equal?(x="Both directions", y=w220) -> (x = y?=w218:bool)
            n132 = Not(x=w218) -> (.not. x?=w219:bool)
            n133 = property on="Rev/Fwd" class="Clust (strict)"("Visible"=w218) -> ()  [unwired: 2 in, 2 out]
            n134 = property on="On/Off" class="Bool (strict)"("Visible"=w219, "Caption.Text"=w217) -> ()  [unwired: 2 in, 2 out]
          }
          frame "Compressor", "Digital Out" {
            w225 = FALSE ("Visible")
            # "Get direction and finish"
            n135 = property on="Motor" class="Clust (strict)"("Visible"=w225) -> ()  [unwired: 2 in, 2 out]
            n136 = property on="Test Slider" class="Slide (strict)"("Visible"=w225) -> ()  [unwired: 2 in, 2 out]
            n137 = property on="Test Ring" class="Ring (strict)"("Visible"=w225) -> ()  [unwired: 2 in, 2 out]
            n138 = property on="On/Off" class="Bool (strict)"("Visible"=TRUE, "Caption.Text"=w226) -> ()  [unwired: 2 in, 2 out]
            n139 = property on="Rev/Fwd" class="Clust (strict)"("Visible"=FALSE) -> ()  [unwired: 2 in, 2 out]
          }
          frame "Camera" {
            n140 = call <vilib>:"NT_Get Last Path Segment.vi"("String in"=w233) -> ("String out"=w234:string)  [unwired: 10 in]
            n141 = property on="On/Off" class="Bool (strict)"("Visible"=FALSE) -> ()  [unwired: 2 in, 2 out]
            n142 = property on="Motor" class="Clust (strict)"("Visible"=FALSE) -> ()  [unwired: 2 in, 2 out]
            n143 = property on="Rev/Fwd" class="Clust (strict)"("Visible"=FALSE) -> ()  [unwired: 2 in, 2 out]
            n144 = case shown="\"White Balance  **\"" w234 {
              tunnel: w233 -> [w240 w249 w258 w267 w276 _ w282]
              tunnel: w232 -> [w238 w246 w255 w264 w273 _ _]
              frame "Size  **" {
                n145 = Index Array(array=w238) -> (element=w237:cluster{string[]})  [unwired: 1 in]
                n146 = call <vilib>:"NT Read String.vi"("name"=w240) -> ("value"=w239:string)  [unwired: 8 in, 2 out]
                n147 = Unbundle(w237) -> (w235:string[])
                n148 = Match First String(2:w235, 3:w239) -> (0:w236:i32)  [unwired: 1 out]
                n149 = property on="Test Ring" class="Ring (strict)"("Value"=w236, "Strings []"=w235) -> ()  [unwired: 2 in, 2 out]
                n150 = property on="Test Ring" class="Ring (strict)"("Visible"=TRUE) -> ()  [unwired: 2 in, 2 out]
                n151 = property on="Test Slider" class="Slide (strict)"("Visible"=FALSE) -> ()  [unwired: 2 in, 2 out]
              }
              frame "White Balance  **" {
                n152 = Index Array(array=w246, index=1) -> (element=w247:cluster{string[]})
                n153 = call <vilib>:"NT Read String.vi"("name"=w249) -> ("value"=w248:string)  [unwired: 8 in, 2 out]
                n154 = Unbundle(w247) -> (w244:string[])
                n155 = Match First String(2:w244, 3:w248) -> (0:w243:i32)  [unwired: 1 out]
                n156 = property on="Test Ring" class="Ring (strict)"("Value"=w243, "Strings []"=w244) -> ()  [unwired: 2 in, 2 out]
                n157 = property on="Test Ring" class="Ring (strict)"("Visible"=TRUE) -> ()  [unwired: 2 in, 2 out]
                n158 = property on="Test Slider" class="Slide (strict)"("Visible"=FALSE) -> ()  [unwired: 2 in, 2 out]
              }
              frame "Exposure  **" {
                n159 = Index Array(array=w255, index=2) -> (element=w256:cluster{string[]})
                n160 = call <vilib>:"NT Read String.vi"("name"=w258) -> ("value"=w257:string)  [unwired: 8 in, 2 out]
                n161 = Unbundle(w256) -> (w252:string[])
                n162 = Match First String(2:w252, 3:w257) -> (0:w253:i32)  [unwired: 1 out]
                n163 = property on="Test Ring" class="Ring (strict)"("Value"=w253, "Strings []"=w252) -> ()  [unwired: 2 in, 2 out]
                n164 = property on="Test Ring" class="Ring (strict)"("Visible"=TRUE) -> ()  [unwired: 2 in, 2 out]
                n165 = property on="Test Slider" class="Slide (strict)"("Visible"=FALSE) -> ()  [unwired: 2 in, 2 out]
              }
              frame "Exposure Priority  **" {
                n166 = Index Array(array=w264, index=3) -> (element=w265:cluster{string[]})
                n167 = call <vilib>:"NT Read String.vi"("name"=w267) -> ("value"=w266:string)  [unwired: 8 in, 2 out]
                n168 = Unbundle(w265) -> (w261:string[])
                n169 = Match First String(2:w261, 3:w266) -> (0:w262:i32)  [unwired: 1 out]
                n170 = property on="Test Ring" class="Ring (strict)"("Value"=w262, "Strings []"=w261) -> ()  [unwired: 2 in, 2 out]
                n171 = property on="Test Ring" class="Ring (strict)"("Visible"=TRUE) -> ()  [unwired: 2 in, 2 out]
                n172 = property on="Test Slider" class="Slide (strict)"("Visible"=FALSE) -> ()  [unwired: 2 in, 2 out]
              }
              frame "Color Enable  **" {
                n173 = Index Array(array=w273, index=4) -> (element=w274:cluster{string[]})
                n174 = call <vilib>:"NT Read String.vi"("name"=w276) -> ("value"=w275:string)  [unwired: 8 in, 2 out]
                n175 = Unbundle(w274) -> (w270:string[])
                n176 = Match First String(2:w270, 3:w275) -> (0:w271:i32)  [unwired: 1 out]
                n177 = property on="Test Ring" class="Ring (strict)"("Value"=w271, "Strings []"=w270) -> ()  [unwired: 2 in, 2 out]
                n178 = property on="Test Ring" class="Ring (strict)"("Visible"=TRUE) -> ()  [unwired: 2 in, 2 out]
                n179 = property on="Test Slider" class="Slide (strict)"("Visible"=FALSE) -> ()  [unwired: 2 in, 2 out]
              }
              frame Default {
                n180 = property on="Test Ring" class="Ring (strict)"("Visible"=FALSE) -> ()  [unwired: 2 in, 2 out]
                n181 = property on="Test Slider" class="Slide (strict)"("Visible"=FALSE) -> ()  [unwired: 2 in, 2 out]
              }
              frame "Brightness  **", "Color Level  **", "Compression  **", "FPS  **", "Sharpness  **" {
                n182 = call <vilib>:"NT Read Number.vi"("name"=w282) -> ("value"=w281:dbl)  [unwired: 8 in, 2 out]
                n183 = local write "Test Slider"(w281) -> ()
                n184 = property on="Test Slider" class="Slide (strict)"("Visible"=TRUE, "Scale.Maximum"=100.0 ("Scale.Range:Maximum")) -> ()  [unwired: 2 in, 2 out]
                n185 = property on="Test Ring" class="Ring (strict)"("Visible"=FALSE) -> ()  [unwired: 2 in, 2 out]
              }
            }
          }
        }
        n186 = property on="Progress" class="Clust (strict)"("Visible"=FALSE) -> ()  [unwired: 2 in, 2 out]
      }
      event "Test Name": Mouse Enter {
        # "Populate the ring with the list of tests"
        n187 = event-data() -> ()  [unwired: 1 in, 1 out]
        n188 = call <vilib>:"NT Read String Array.vi"("name"="TestMode/TestList" ("Name")) -> ("value"=w289:string[])  [unwired: 8 in, 2 out]
        n189 = Build Array (concatenate)("Select the test to run...", w289) -> (w288:string[])
        n190 = property on="Test Name" class="Ring (strict)"("Strings []"=w288) -> ()  [unwired: 2 in, 2 out]
      }
      event "Test Name": Value Change {
        w290 = FALSE ("Visible")
        # "Tell the robot the test name to run"
        n191 = event-data() -> ("NewVal"=w294:u16)  [unwired: 1 in]
        n192 = property on="Test Name" class="Ring (strict)"() -> ("Strings []"=w295:string[])  [unwired: 2 in, 2 out]
        n193 = local write "Progress"(T6 {"Test Progress"=0, "Test Progress Text"=""} ("Progress")) -> ()
        n194 = Index Array(array=w295, index=w294) -> (element=w293:string)
        n195 = call <vilib>:"NT Write String.vi"("value"=w293, "name"="TestMode/TestName" ("Name")) -> ()  [unwired: 9 in, 1 out]
        n196 = property on="Progress" class="Clust (strict)"("Visible"=TRUE) -> ()  [unwired: 2 in, 2 out]
        n197 = property on="Motor" class="Clust (strict)"("Visible"=w290) -> ()  [unwired: 2 in, 2 out]
        n198 = property on="Test Slider" class="Slide (strict)"("Visible"=w290) -> ()  [unwired: 2 in, 2 out]
        n199 = property on="On/Off" class="Bool (strict)"("Visible"=w290) -> ()  [unwired: 2 in, 2 out]
        n200 = property on="Rev/Fwd" class="Clust (strict)"("Visible"=w290) -> ()  [unwired: 2 in, 2 out]
        n201 = property on="Test Ring" class="Ring (strict)"("Visible"=w290) -> ()  [unwired: 2 in, 2 out]
      }
      event "Select Auto": Mouse Enter {
        # "Populate the combo box with the list of autonomous options"
        n202 = event-data() -> ()  [unwired: 1 in, 1 out]
        n203 = call <vilib>:"NT Read String Array.vi"("name"="Auto List" ("Name")) -> ("value"=w297:string[])  [unwired: 8 in, 2 out]
        n204 = property on="Select Auto" class="CmbBox"("Strings[]"=w297) -> ()  [unwired: 2 in, 2 out]
      }
      event "Select Auto": Value Change {
        # "User modified the Auto Selection. Write to NT variable so robot knows."
        n205 = event-data() -> ("NewVal"=w299:string)  [unwired: 1 in]
        n206 = call <vilib>:"NT Write String.vi"("value"=w299, "name"="Auto Selector" ("Name")) -> ()  [unwired: 9 in, 1 out]
      }
      event "CheckList": Double Click {
        # "Shift clears all"
        # "Update symbols on the listbox"
        n207 = event-data() -> ("PlatMods.Shift"=w301:bool, "Row"=w303:i32)  [unwired: 1 in]
        n208 = case shown="True" w301 {
          tunnel: w303 -> [w307 _]
          tunnel: 1 -> [w306 _]
          frame False {
            n209 = property on="CheckList" class="LstBox (strict)"() -> ("Item Symbols"=w305:i32[])  [unwired: 2 in, 2 out]
            n210 = Replace Array Subset(array=w305, new element=w306, index=w307) -> (w304:i32[])
            n211 = property on="CheckList" class="LstBox (strict)"("Item Symbols"=w304) -> ()  [unwired: 2 in, 2 out]
          }
          frame True {
            w308 = 0 ("Top Row")
            n212 = property on="CheckList" class="LstBox (strict)"() -> ("Number of Rows"=w310:u32)  [unwired: 2 in, 2 out]
            n213 = Initialize Array(0, w310) -> (w309:i32[])
            n214 = property on="CheckList" class="LstBox (strict)"("Top Row"=w308, "Value"=w308, "Item Symbols"=w309) -> ()  [unwired: 2 in, 2 out]
          }
        }
      }
      event "CheckList": Key Down {
        # "Update symbols on the listbox\nLeft and right keys check and uncheck"
        n215 = event-data() -> ("VKey"=w313:T14)  [unwired: 1 in]
        n216 = case shown="\"Left\", \"Right\"" w313 {
          selector: w313 -> [w318 _]
          tunnel: eventvkey."Left" ("VKey") -> [w316 _]
          frame "Left", "Right" {
            n217 = Equal?(x=w316, y=w318) -> (x = y?=w317:bool)
            n218 = Select(t=0, s=w317, f=1) -> (s? t:f=w319:i32)
            n219 = property on="CheckList" class="LstBox (strict)"() -> ("Item Symbols"=w322:i32[])  [unwired: 2 in, 2 out]
            n220 = Replace Array Subset(array=w322, new element=w319, index="CheckList") -> (w321:i32[])
            n221 = property on="CheckList" class="LstBox (strict)"("Item Symbols"=w321) -> ()  [unwired: 2 in, 2 out]
          }
          frame Default {
          }
        }
      }
      event "Motor.Enable": Value Change {
        # "When the test mode otor enable helper is set, update that\ntree row item's value"
        n222 = event-data() -> ("NewVal"=w327:bool)  [unwired: 1 in]
        n223 = Unbundle("Motor") -> ("Value"=w326:dbl)  [unwired: 1 out]
        n224 = Select(t=w326, s=w327, f=0.0) -> (s? t:f=w324:dbl)
        n225 = call <vilib>:"NT Write Number.vi"("value"=w324, "name"=w323) -> ()  [unwired: 9 in, 1 out]
      }
      event "Test Slider": Value Change {
        # "When the test mode slider helper is set, update that\ntree row item's value"
        n226 = event-data() -> ("NewVal"=w329:dbl)  [unwired: 1 in]
        n227 = call <vilib>:"NT Write Number.vi"("value"=w329, "name"=w330) -> ()  [unwired: 9 in, 1 out]
      }
      event "On/Off": Value Change {
        # "When the test mode on/off helper value is set, update that\ntree row item's value"
        n228 = event-data() -> ("NewVal"=w333:bool)  [unwired: 1 in]
        n229 = Boolean To (0,1)(Boolean=w333) -> (0, 1=w332:i16)
        n230 = call <vilib>:"NT Write Number.vi"("value"=w332, "name"=w331) -> ()  [unwired: 9 in, 1 out]
      }
      event "Rev/Fwd": Value Change {
        # "When the test mode helper value for relays is set, update that\ntree row item's value"
        n231 = event-data() -> ("NewVal.Forward"=w340:bool, "NewVal.Reverse"=w339:bool)  [unwired: 1 in]
        n232 = Boolean To (0,1)(Boolean=w340) -> (0, 1=w336:i16)
        n233 = Boolean To (0,1)(Boolean=w339) -> (0, 1=w338:i16)
        n234 = Negate(x=w338) -> (-x=w337:i16)
        n235 = Add(x=w336, y=w337) -> (x+y=w335:i16)
        n236 = call <vilib>:"NT Write Number.vi"("value"=w335, "name"=w334) -> ()  [unwired: 9 in, 1 out]
      }
      event "Test Ring": Value Change {
        # "When a test mode helper value is selected from the ring,\nset the tree item's variable to the string value"
        n237 = event-data() -> ("NewVal"=w343:u16)  [unwired: 1 in]
        n238 = property on="Test Ring" class="Ring (strict)"() -> ("Strings []"=w344:string[])  [unwired: 2 in, 2 out]
        n239 = Index Array(array=w344, index=w343) -> (element=w342:string)
        n240 = call <vilib>:"NT Write String.vi"("value"=w342, "name"=w341) -> ()  [unwired: 9 in, 1 out]
      }
      event "Rec Mode": Value Change {
        # "Update globals for recording mode and path to read log from.\nClear when logging and let NetworkTables set path for vision to\nuse."
        n241 = event-data() -> ("NewVal"=w353:enum32{"Stop", "Record", "Playback"})  [unwired: 1 in]
        n242 = global write "WPI_DashboardLogging Global.vi" "Logging Filename"(path "") -> ()
        n243 = global write "WPI_DashboardLogging Global.vi" "Recording"(w353) -> ()
        n244 = case shown="\"Playback\"" w353 {
          tunnel: w352 -> [_ w355 w363]
          tunnel: [_ _ w362] -> w350
          tunnel: [_ _ w361] -> _
          tunnel: w348 -> [_ _ w359]
          tunnel: cluster{i32, i32} {-250, 170} -> [_ _ w358]
          tunnel: [_ _ T15 {"Image Size"=TRUE, "Image Type"=TRUE, "Pixel Value"=TRUE, "ROI Information"=TRUE, "Zoom Factor"=FALSE} ("Image Information Shown:All Elements")] -> w345
          tunnel: [_ _ TRUE ("Zoom Factor")] -> w346
          frame Default {
          }
          frame "Stop", "Record" {
            # "Place Window too"
            n245 = invoke class="VI" method="FP.Close"(reference=w355) -> (reference out=w354:refnum<vi>)  [unwired: 2 in, 2 out]
            n246 = invoke class="VI" method="Abort VI"(reference=w354) -> ()  [unwired: 2 in, 3 out]
          }
          frame "Playback" {
            n247 = call "Open Playback Panel.vi"("Offset"=w358, "DB VI Ref"=w359, "Playback in"=w363) -> ("Playback out"=w360:refnum<vi>)  [unwired: 8 in]
            n248 = register-events(w360) -> (reference out=w362:refnum<event-registration>, error out=w361:errorcluster)  [unwired: 2 in]
          }
        }
        n249 = property on="Camera Image Right" class="ImageControl"("Image Information Shown"=w345, "Image Information Visible"=w346) -> ()  [unwired: 2 in, 2 out]
        n250 = property on="Camera Image" class="ImageControl"("Image Information Shown"=w345, "Image Information Visible"=w346) -> ()  [unwired: 2 in, 2 out]
        n251 = call <vilib>:"WPI_DashboardNT Log FieldName Cache.vi"("Operation"=enum16{"Lookup/Add", "Index", "Clear"}."Clear") -> ()  [unwired: 8 in, 3 out]
      }
      event Panel Close {
        w364 = enum32{"Stop", "Record", "Playback"}."Stop" ("Rec Mode")
        # "Playback window has been closed, abort"
        n252 = event-data() -> ()  [unwired: 1 in, 4 out]
        n253 = local write "Rec Mode"(w364) -> ()
        n254 = global write "WPI_DashboardLogging Global.vi" "Recording"(w364) -> ()
      }
      event Panel Close {
        # "Abort playback window and ourself"
        n255 = event-data() -> ()  [unwired: 1 in, 4 out]
        n256 = invoke class="VI" method="FP.Close"(reference=w367) -> (reference out=w366:refnum<vi>)  [unwired: 2 in, 2 out]
        n257 = invoke class="VI" method="Abort VI"(reference=w366) -> (error out=w365:errorcluster)  [unwired: 2 in, 2 out]
        n258 = invoke class="VI" method="Abort VI"(error in=w365) -> ()  [unwired: 2 in, 3 out]
      }
      event "Tree": Double Click {
        n259 = event-data() -> ("PlatMods"=w373:T17, "Tag"=w370:string)  [unwired: 1 in]
        n260 = Unbundle(w373) -> ("Shift"=w372:bool)  [unwired: 4 out]
        n261 = String Subset(string=w370, length (rest)=1 ("length (rest)")) -> (substring=w369:string)  [unwired: 1 in]
        n262 = Not(x=w372) -> (.not. x?=w371:bool)
        n263 = case shown="\"/\"" w369 {
          tunnel: w370 -> [_ w375]
          tunnel: w371 -> [_ w374]
          frame Default {
          }
          frame "/" {
            n264 = call <vilib>:"NT Update Persistence.vi"("Persistence"=w374, "Name"=w375) -> ()  [unwired: 9 in, 1 out]
          }
        }
      }
    }
  }
  n265 = while {
    tunnel: [w384] -> _
    tunnel: w25 -> [w376]
    i -> [w384]
    stop <- FALSE stop-if-true
    n266 = call <vilib>:"WPI_DashboardRetrieveStatusInfo.vi"("Window Mode Notifier"=w376, "TCP Cnx"="TCP") -> ("Power and Errors"=w379:T18, "Robot Metrics"=w382:T19, "Status Info"=w383:T20, "Control Info"=w380:T21, "Robot Mode"=w378:T4, "Process?"=w381:bool)  [unwired: 4 in]
    "Mode" <- w378
    n267 = case shown="True" w381 {
      tunnel: w383 -> [_ w410]
      tunnel: w382 -> [_ w409]
      tunnel: w380 -> [_ w408]
      tunnel: w379 -> [_ w407]
      tunnel: w378 -> [_ _]
      frame False {
        n268 = Wait (ms)(milliseconds to wait=u32 20) -> ()  [unwired: 1 out]
      }
      frame True {
        # "swap motors to match\ncharts and include battery"
        n269 = Unbundle By Name(w408) -> ("Joystick Values"=w398:T22)  [unwired: 1 out]
        n270 = Unbundle By Name(w409) -> ()  [unwired: 1 out]
        n271 = Unbundle By Name(w407) -> ("Robot IP"=→"Robot IP":string)
        n272 = Unbundle By Name(w410) -> ()  [unwired: 2 out]
        n273 = call-poly <vilib>:"NT Read Value.vi"("name"="RobotDrive Motors" ("Name")) -> ("value"=w388:dbl[])  [unwired: 8 in, 2 out]
        n274 = Index Array(array=w388, index #1=1, index #4=0) -> (element #1=w402:dbl, element #2=w403:dbl, element #3=w401:dbl, element #4=w406:dbl)  [unwired: 2 in]
        n275 = Index Array(array=w398) -> (element #1=w397:T23, element #2=w393:T23)  [unwired: 2 in]
        n276 = call "Prepare Joystick Data for Displays.vi"("Joystick Values"=w393) -> ("Buttons"=→"JS2 Buttons":T24, "Z Axis"=→"JS2 Z":dbl, "Cartesian Data"=→"JS2 Graph":cluster{"X axis":dbl, "X axis":dbl}[])  [unwired: 8 in]
        n277 = call "Prepare Joystick Data for Displays.vi"("Joystick Values"=w397) -> ("Buttons"=→"JS1 Buttons":T24, "Z Axis"=→"JS1 Z":dbl, "Cartesian Data"=→"JS1 Graph":cluster{"X axis":dbl, "X axis":dbl}[])  [unwired: 8 in]
        n278 = Bundle("Numeric"=w401, "Numeric"=w402) -> (→"MotorChart R" →"MotorSliders R":cluster{"Numeric":dbl, "Numeric":dbl})  [unwired: 1 in]
        n279 = Bundle("Numeric"=w403, "Numeric"=w406) -> (→"MotorChart L" →"MotorSliders L":cluster{"Numeric":dbl, "Numeric":dbl})  [unwired: 1 in]
      }
    }
  }
  n280 = while {
    tunnel: w61 -> [w424]
    tunnel: w60 -> [_]
    tunnel: w3 -> [w417]
    tunnel: w1 -> [w414]
    stop <- FALSE stop-if-true
    # "Optionally read the DB image,\nlog, or retrieve images from a\nlogged match"
    n281 = local read "NT Connection"() -> (w418:bool)
    n282 = local read "Rec Mode"() -> (w421:enum32{"Stop", "Record", "Playback"})
    n283 = local read "Right Camera Perf"() -> (w412:cluster{"Bandwidth (Mbps)":dbl, "FPS":dbl})
    n284 = Bundle("Camera Name"="Camera Name", w414, "Saved DB Images Info"=w417) -> (w416:T25)  [unwired: 1 in]
    n285 = control-ref of="Camera Perf"() -> (w411:refnum<vi>)
    n286 = call <vilib>:"WPI_CameraRead MJPG for Dashboard_2.vi"("Camera Settings"="Camera Settings", "Rec Mode"=w421, "NT Connection"=w418, "Capture Info"=w416, "Image in"=w424) -> ("perf info"=w413:cluster{"Bandwidth (Mbps)":dbl, "fps":dbl}, "Active"=w422:bool, "Image\\ out"=w423:T5)  [unwired: 4 in]
    n287 = case shown="True" w422 {
      tunnel: w423 -> [w427 w430]
      tunnel: [w427 w429] -> w419
      frame False {
        # "Sleep for 500ms"
        n288 = property on="Camera Image" class="ImageControl"("ROI"=T11 {"Global Rectangle"=[], "Contours"=[]}) -> ()  [unwired: 2 in, 2 out]
        n289 = Wait Until Next ms Multiple(millisecond multiple=u32 500) -> ()  [unwired: 1 out]
      }
      frame True {
        # "Here is where you would annotate,\npossibly process, and display the image"
        # "Update Mbps LED"
        n290 = call "IMAQ Clear Overlay"("Image"=w430) -> ("error out"=w431:errorcluster, "Image Out"=w429:T5)  [unwired: 2 in, 7 out]
        n291 = Unbundle By Name(w431) -> ("status"=w432:bool)
        n292 = property on="Image Message" class="Str"("Visible"=w432) -> ()  [unwired: 2 in, 2 out]
      }
    }
    "Camera Image" <- w419
    n293 = call <vilib>:"WPI_DashboardFormatPerf.vi"("Right Camera Perf"=w412, "Performance"=w413, "String in"=w411) -> ()  [unwired: 9 in]
  }
  n294 = while {
    tunnel: w54 -> [w434]
    i -> [w437]
    stop <- FALSE stop-if-true
    n295 = Wait (ms)(milliseconds to wait=u32 100) -> ()  [unwired: 1 out]
    n296 = case shown="\"Playback\"" "Rec Mode" {
      tunnel: w437 -> [_ _ w452]
      tunnel: [u32 2829099 ("Base Color") u32 11141120 ("Target Color") w441] -> w433
      frame "Stop", Default {
        # "Reset the color, extra updates don't cost much"
      }
      frame "Record" {
      }
      frame "Playback" {
        # "Playback"
        n297 = Quotient & Remainder(x=w452, y=u32 50 ("milliseconds to wait")) -> (x-y*floor(x/y)=w448:u32)  [unwired: 1 out]
        n298 = Divide(x=w448, y=u32 50 ("milliseconds to wait")) -> (x/y=w445:dbl)
        n299 = Multiply(x=6.283185307179586, y=w445) -> (x*y=w450:dbl)
        n300 = Sine(x=w450) -> (sin(x)=w449:dbl)
        n301 = Absolute Value(x=w449) -> (abs(x)=w442:dbl)
        n302 = call "Interpolate RGB Color.vi"("Proportion"=w442, "Target Color"=u32 30976, "Base Color"=u32 2829099) -> ("Result Color"=w441:u32)  [unwired: 8 in]
      }
    }
    n303 = property class="Pane"(reference=w434, "PaneColor"=w433) -> ()  [unwired: 1 in, 2 out]
  }
  n304 = local write "Dashboard Tab"(T2."Drive" ("Dashboard Tab")) -> ()
  n305 = property on="On/Off" class="Bool (strict)"("Visible"=w26) -> ()  [unwired: 2 in, 2 out]
  n306 = property on="Motor" class="Clust (strict)"("Visible"=w26) -> ()  [unwired: 2 in, 2 out]
  n307 = property on="Progress" class="Clust (strict)"("Visible"=w26) -> ()  [unwired: 2 in, 2 out]
  n308 = property on="Test Ring" class="Ring (strict)"("Visible"=w26) -> ()  [unwired: 2 in, 2 out]
  n309 = property on="Rev/Fwd" class="Clust (strict)"("Visible"=w26) -> ()  [unwired: 2 in, 2 out]
  n310 = while {
    tunnel: u16 1741 ("timeout ms (25000)") -> [w454]
    stop <- FALSE stop-if-true
    n311 = TCP Create Listener(10:w454) -> (0:w453:errorcluster, 3:w455:refnum<k5>)  [unwired: 4 in, 1 out]
    n312 = case shown="No Error" w453 {
      selector: w453 -> [w457 _]
      tunnel: w455 -> [w458 _]
      frame No Error {
        n313 = while {
          tunnel: w458 -> [w461]
          tunnel: w457 -> [w460]
          stop <- FALSE stop-if-true
          n314 = TCP Wait On Listener(8:w460, 11:w461) -> (0:w462:errorcluster, 4:w463:refnum<k5>)  [unwired: 2 in, 3 out]
          n315 = local write "TCP"(w463) -> ()
          n316 = case shown="Error" w462 {
            frame No Error {
            }
            frame Error {
              n317 = Wait (ms)(milliseconds to wait=u32 1000) -> ()  [unwired: 1 out]
            }
          }
        }
      }
      frame Error {
        n318 = Wait (ms)(milliseconds to wait=u32 1000) -> ()  [unwired: 1 out]
      }
    }
  }
  n319 = global write "WPI_DashboardLogging Global.vi" "Recording"(w49) -> ()
  n320 = local write "Rec Mode"(w49) -> ()
  n321 = call <vilib>:"NT Write String.vi"("value"="Select Auto", "name"="Auto Selector" ("Name")) -> ()  [unwired: 9 in, 1 out]
